vi "LV_File_Stop.vi"(8 "error in":errorcluster, 11 "LV_File.lvclass (IN)":refnum<class "LV_File.lvclass">) -> (0 "error out":errorcluster, 3 "LV_File.lvclass (OUT)":refnum<class "LV_File.lvclass">)   [LabVIEW 2013, in "LV_File.lvclass"]
uses:
  LV_File.lvclass
  LV_File.lvclass/LV_File.ctl
  File.lvclass
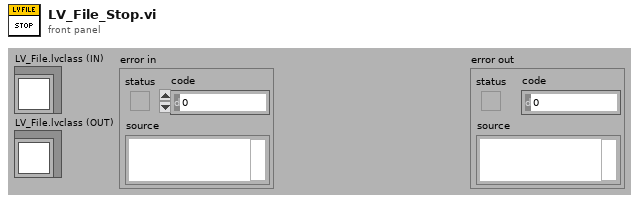
[diagram p1: front panel]
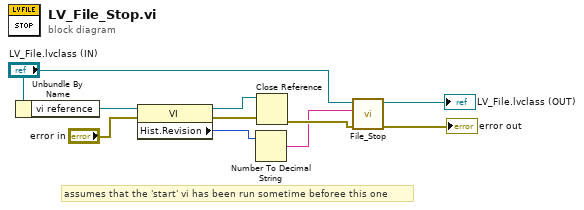
[diagram p0: block diagram]
diagram:
  # "assumes that the 'start' vi has been run sometime beforee this one"
  n1 = Unbundle By Name("LV_File.lvclass (IN)") -> ("vi reference"=w7:refnum<vi>)
  n2 = property class="VI"(reference=w7, error in="error in") -> (reference out=w6:refnum<vi>, error out=w8:errorcluster, "Hist.Revision"=w3:u32)
  n3 = Number To Decimal String(number=w3) -> (decimal integer string=w2:string)  [unwired: 1 in]
  n4 = Close Reference(reference=w6, error in (no error)=w8) -> (error out=w5:errorcluster)
  n5 = call "File_Stop.vi"("error in"=w5, "Version"=w2, "File.lvclass (IN)"="LV_File.lvclass (IN)") -> ("error out"=→"error out":errorcluster, "File.lvclass (OUT)"=→"LV_File.lvclass (OUT)":refnum<class "LV_File.lvclass">)  [unwired: 7 in]
